vi "Class.Unflatten.vi"(8 "error in":errorcluster, 11 "Flattened Class":string) -> (0 "error out":errorcluster, 3 "Data Access API":refnum<class "Data Access API.lvclass">)   [LabVIEW 2015, in "Data Access API.lvlib" / "Data Access API.lvclass"]
uses:
  Data Access API.lvclass
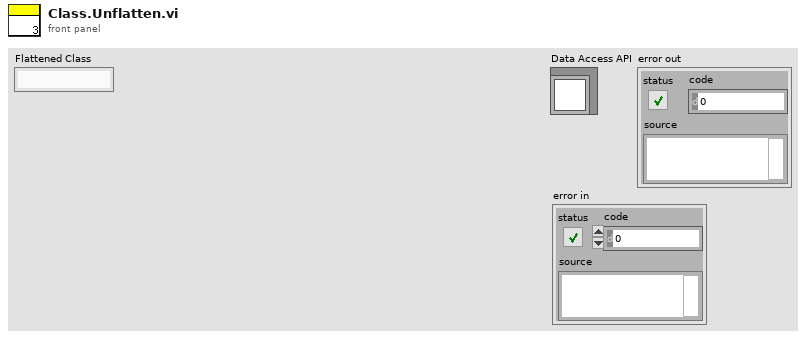
[diagram p1: front panel]
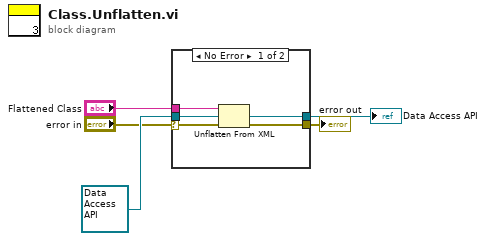
[diagram p0: block diagram]
diagram:
  n1 = case shown="No Error" "error in" {
    selector: "error in" -> [w7 w12]
    tunnel: "Flattened Class" -> [w10 _]
    tunnel: refnum<class "Data Access API.lvclass"> refnum ("Data Access API.lvlib:Data Access API.lvclass") -> [w9 w11]
    tunnel: [w8 w11] -> w3
    tunnel: [w6 w12] -> w2
    frame No Error {
      n2 = Unflatten From XML(xml string=w10, type=w9, error in (no error)=w7) -> (value=w8:refnum<class "Data Access API.lvclass">, error out=w6:errorcluster)
    }
    frame Error {
    }
  }
  "Data Access API" <- w3
  "error out" <- w2
